vi "Value_Occurence_Analysis.vi"(3 "Average Numeric Values?":bool, 4 "Tolerance":dbl=1.0 format="%.2f", 5 "Precision (3)":string, 6 "String Array":string[](array[string])) -> (0 "Numeric Array?":bool, 1 "St Dev":string, 2 "Output String":string)   [LabVIEW 2020]
uses:
  <vilib>/Analysis/NI_AALBase.lvlib
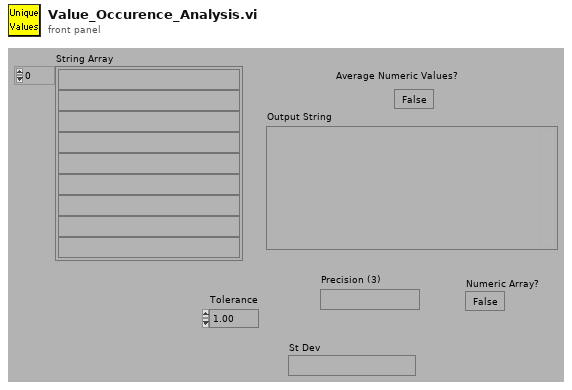
[diagram p1: front panel]
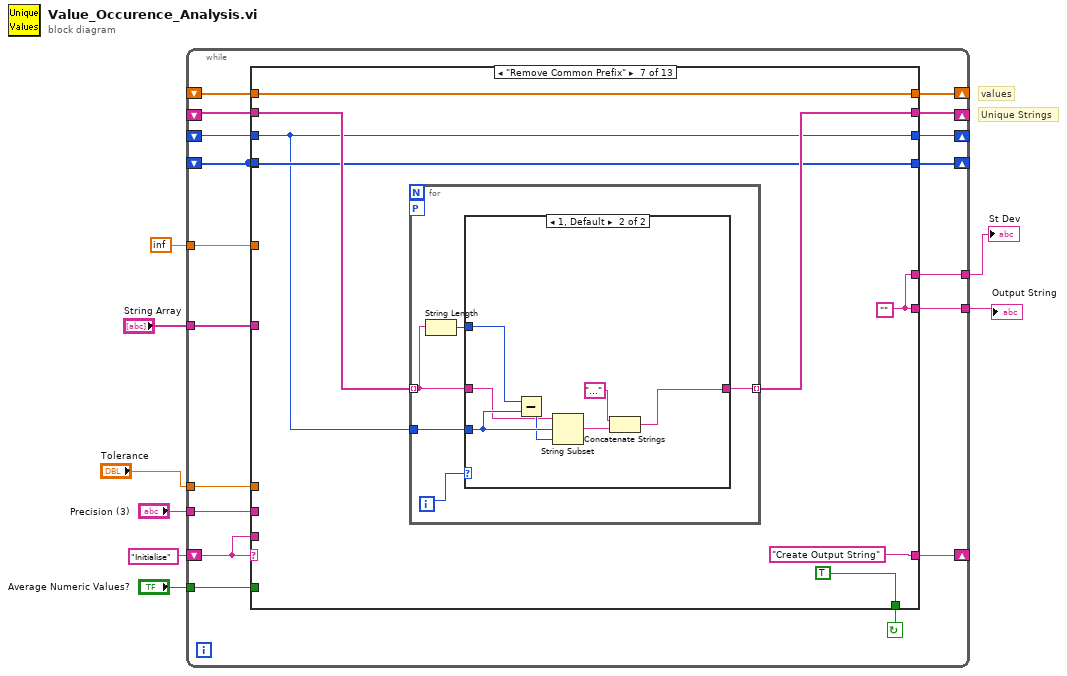
[diagram p0: block diagram]
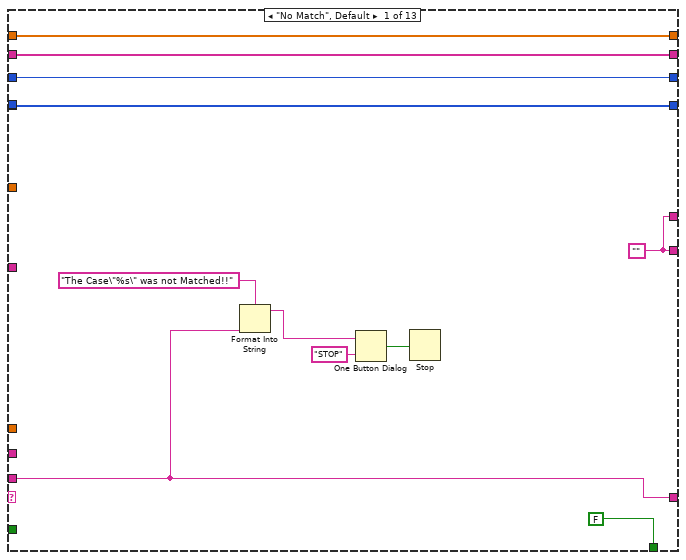
[diagram p2: hidden frame]
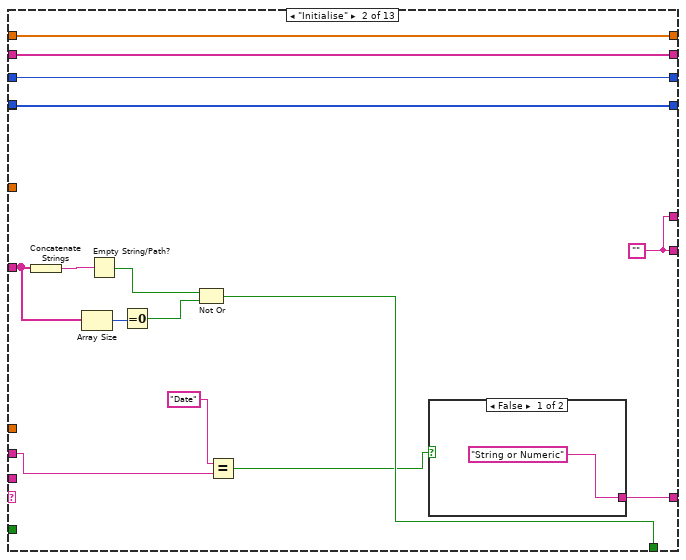
[diagram p3: hidden frame]
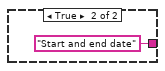
[diagram p4: hidden frame]
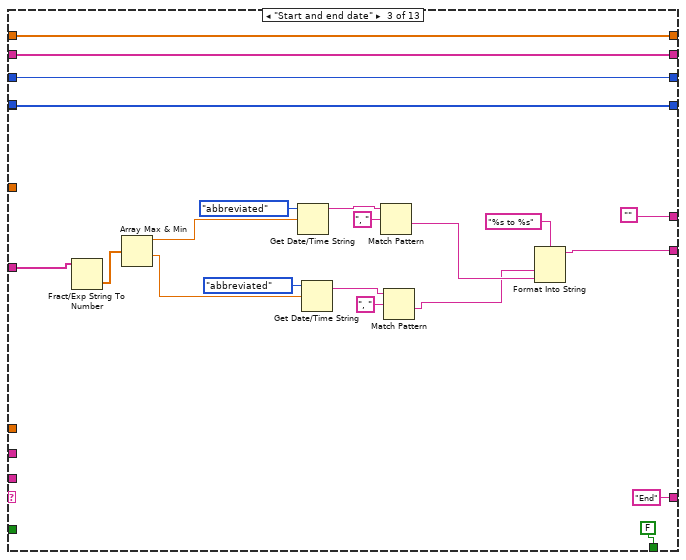
[diagram p5: hidden frame]
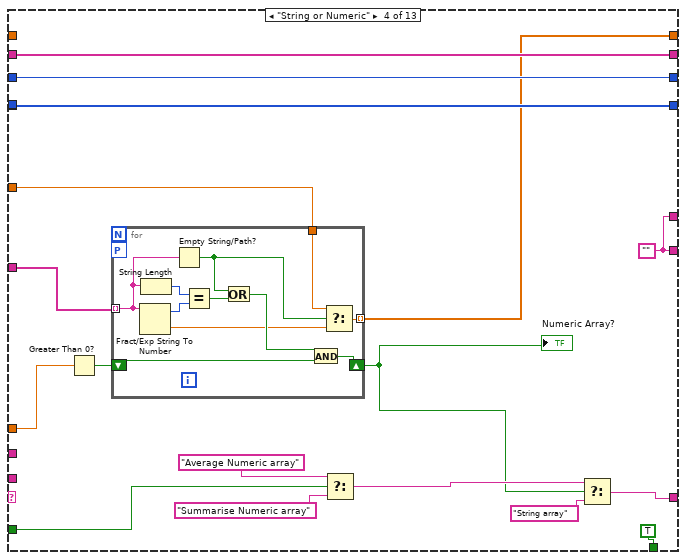
[diagram p6: hidden frame]
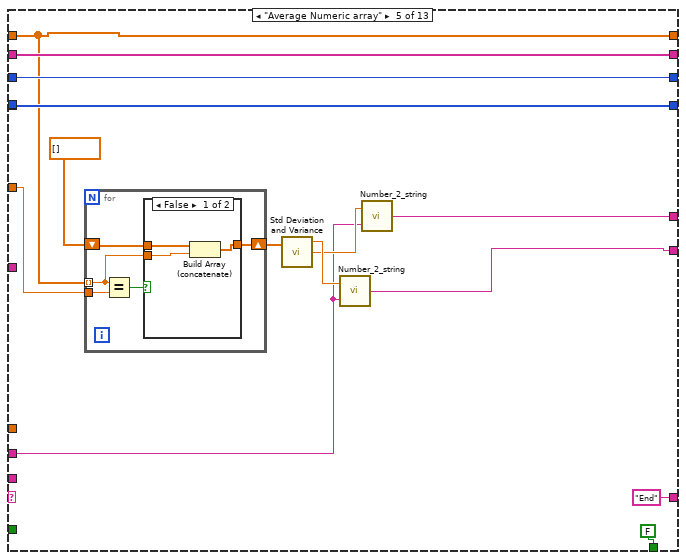
[diagram p7: hidden frame]
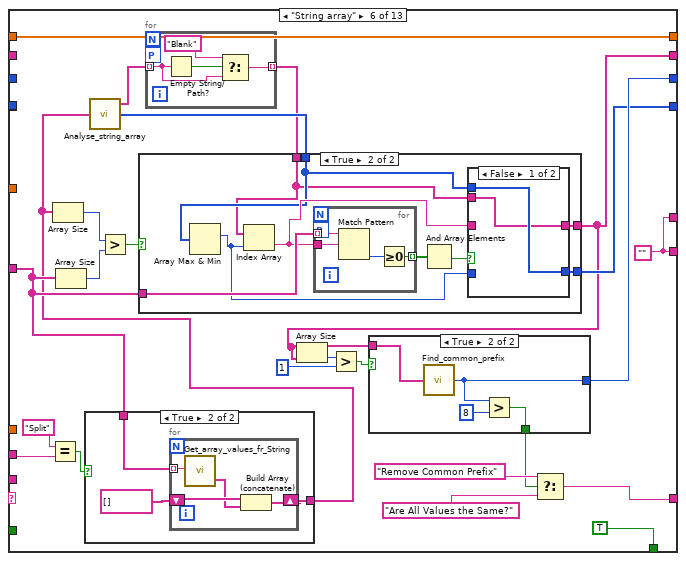
[diagram p9: hidden frame]
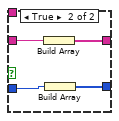
[diagram p12: hidden frame]
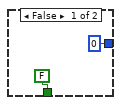
[diagram p13: hidden frame]
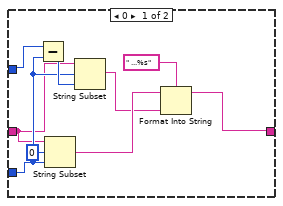
[diagram p14: hidden frame]
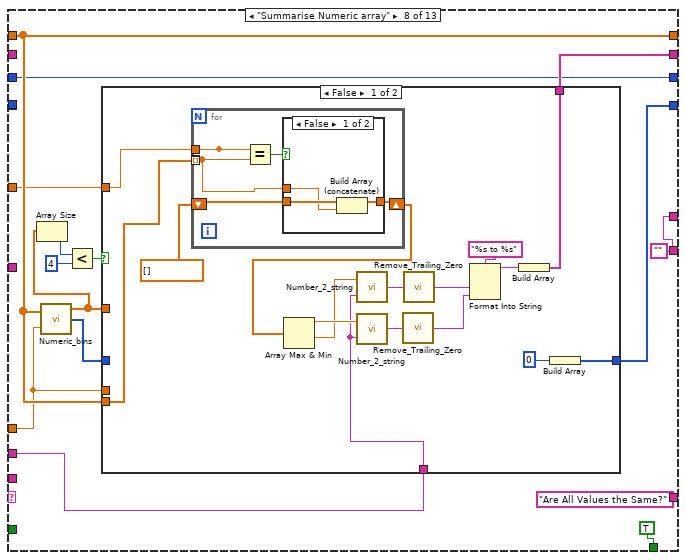
[diagram p15: hidden frame]
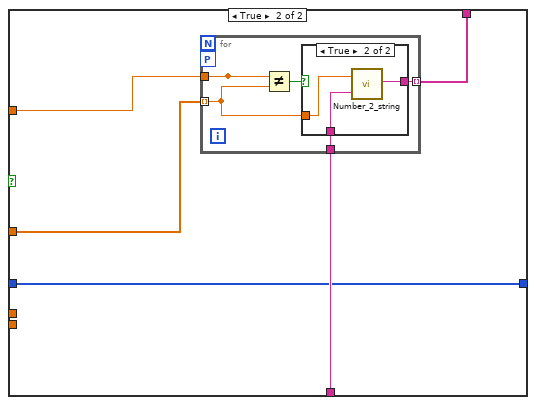
[diagram p17: hidden frame]
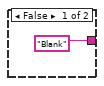
[diagram p18: hidden frame]
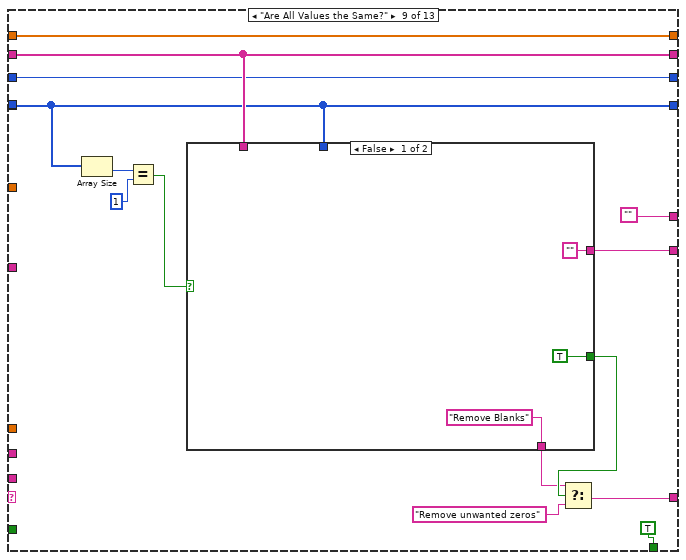
[diagram p19: hidden frame]
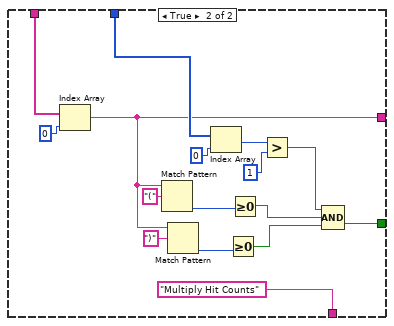
[diagram p20: hidden frame]
diagram:
  # "Unique Strings"
  # "values"
  n1 = while {
    shift-left: _ -> [w12]
    shift-right: [w13] -> _
    tunnel: [w14] -> w6
    shift-left: _ -> [w15]
    shift-right: [w16] -> _
    shift-left: _ -> [w17]
    shift-right: [w18] -> _
    tunnel: "Tolerance" -> [w19]
    shift-left: _ -> [w20]
    shift-right: [w24] -> _
    shift-left: "Initialise" -> [w21]
    shift-right: [w23] -> _
    tunnel: inf -> [w25]
    tunnel: "String Array" -> [w26]
    tunnel: "Average Numeric Values?" -> [w11]
    tunnel: "Precision (3)" -> [w10]
    tunnel: [w9] -> w2
    stop <- w22 continue-if-true
    n2 = case shown="\"Remove Common Prefix\"" w21 {
      tunnel: w26 -> [_ w47 w62 w88 _ w136 _ _ _ _ _ _ _]
      tunnel: w25 -> [_ _ _ w76 w111 _ _ w228 _ _ _ _ _]
      tunnel: [w32 w52 w71 w77 w110 w149 w196 w230 w286 w318 w350 w383 w401] -> w24
      tunnel: [w33 w49 "End" w91 "End" w144 "Create Output String" "Are All Values the Same?" w274 "End" "Remove unwanted zeros" "Create Output String" "Initialise"] -> w23
      tunnel: [FALSE w43 FALSE TRUE FALSE TRUE TRUE TRUE TRUE FALSE TRUE TRUE FALSE] -> w22
      tunnel: w21 -> [w33 _ _ _ _ _ _ _ _ _ _ _ _]
      tunnel: w20 -> [w32 w52 w71 _ w110 w149 w196 w230 w286 w318 w350 w383 w401]
      tunnel: w19 -> [_ _ _ w86 _ _ _ w229 _ _ _ _ _]
      tunnel: [w30 w51 w73 w89 w116 w134 w192 w227 w279 w315 w347 w382 w391] -> w18
      tunnel: w17 -> [w30 w51 w73 w89 w116 _ w192 _ w279 w315 w349 w382 w391]
      tunnel: w17 -> [_ _ _ _ _ _ _ _ _ _ _ _ _]
      tunnel: [w29 w50 w75 w90 w117 w133 w194 w231 w283 w317 w348 w379 w398] -> w16
      tunnel: w15 -> [w29 w50 w75 w90 w117 _ w193 _ w283 w317 w346 w380 w398]
      tunnel: [w27 w41 w65 w78 w112 w140 w190 w219 w281 w309 w344 w378 w397] -> w14
      tunnel: [w28 w42 w74 w84 w114 w148 w191 w222 w282 w316 w345 w381 w396] -> w13
      tunnel: w12 -> [w28 w42 w74 w84 w114 _ w191 w222 w282 w316 w345 w381 w396]
      tunnel: w11 -> [_ _ _ w83 _ _ _ _ _ _ _ _ _]
      tunnel: w10 -> [_ w40 _ _ w105 w132 _ w220 _ _ _ _ _]
      tunnel: [w27 w41 "" w78 w104 w140 w190 w219 "" "" w344 w378 ""] -> w9
      frame "No Match", Default {
        w27 = ""
        n3 = Format Into String(format string="The Case\"%s\" was not Matched!!" ("Format String"), w33) -> (resulting string=w36:string)  [unwired: 2 in, 1 out]
        n4 = One Button Dialog(message=w36, button name ("OK")="STOP") -> (true=w31:bool)
        n5 = Stop(stop? (T)=w31) -> ()
      }
      frame "Initialise" {
        w41 = ""
        n6 = Concatenate Strings(w47) -> (w48:string)
        n7 = Array Size(array=w47) -> (size(s)=w45:i32)
        n8 = Empty String/Path?(string/path=w48) -> (empty?=w46:bool)
        n9 = Equal To 0?(x=w45) -> (x = 0?=w44:bool)
        n10 = Not Or(1:w44, 2:w46) -> (0:w43:bool)
        n11 = Equal?(x="Date", y=w40) -> (x = y?=w38:bool)
        n12 = case shown="False" w38 {
          tunnel: ["String or Numeric" "Start and end date"] -> w49
          frame False {
          }
          frame True {
          }
        }
      }
      frame "Start and end date" {
        n13 = Fract/Exp String To Number(string=w62) -> (number=w61:dbl[])  [unwired: 4 out]
        n14 = Array Max & Min(array=w61) -> (max value=w70:dbl, min value=w67:dbl)  [unwired: 2 out]
        n15 = Get Date/Time String(date format (0)=enum16{"short", "long", "abbreviated"}."abbreviated", seconds (now)=w70) -> (date string=w59:string)  [unwired: 2 out]
        n16 = Get Date/Time String(date format (0)=enum16{"short", "long", "abbreviated"}."abbreviated", seconds (now)=w67) -> (date string=w57:string)  [unwired: 2 out]
        n17 = Match Pattern(string=w59, regular expression=", ") -> (after substring=w56:string)  [unwired: 4 out]
        n18 = Match Pattern(string=w57, regular expression=", ") -> (after substring=w55:string)  [unwired: 4 out]
        n19 = Format Into String(format string="%s to %s", w55, w56) -> (resulting string=w65:string)  [unwired: 2 in, 1 out]
      }
      frame "String or Numeric" {
        w78 = ""
        n20 = Greater Than 0?(x=w86) -> (x > 0?=w85:bool)
        n21 = for {
          tunnel: w88 -> [w94] mode=indexing
          shift-right: [w101] -> w79
          shift-left: w85 -> [w102]
          tunnel: [w98] -> w77 mode=indexing
          tunnel: w76 -> [w99]
          workers-P: _ -> [_]
          n22 = Fract/Exp String To Number(string=w94) -> (offset past number=w96:i32, number=w97:dbl)  [unwired: 3 out]
          n23 = String Length(string=w94) -> (length=w95:i32)
          n24 = Empty String/Path?(string/path=w94) -> (empty?=w100:bool)
          n25 = Equal?(x=w95, y=w96) -> (x = y?=w93:bool)
          n26 = Or(x=w100, y=w93) -> (x .or. y?=w103:bool)
          n27 = And(x=w103, y=w102) -> (x .and. y?=w101:bool)
          n28 = Select(t=w99, s=w100, f=w97) -> (s? t:f=w98:dbl)
        }
        "Numeric Array?" <- w79
        n29 = Select(t="Average Numeric array", s=w83, f="Summarise Numeric array") -> (s? t:f=w80:string)
        n30 = Select(t=w80, s=w79, f="String array") -> (s? t:f=w91:string)
      }
      frame "Average Numeric array" {
        n31 = for {
          shift-right: [w118] -> w108
          shift-left: dbl[] [] -> [w120]
          tunnel: w111 -> [w122]
          tunnel: w110 -> [w119] mode=indexing
          n32 = Equal?(x=w119, y=w122) -> (x = y?=w121:bool)
          n33 = case shown="False" w121 {
            tunnel: w120 -> [w125 w126]
            tunnel: w119 -> [w124 _]
            tunnel: [w123 w126] -> w118
            frame False {
              n34 = Build Array (concatenate)(w125, w124) -> (w123:dbl[])
            }
            frame True {
            }
          }
        }
        n35 = call <vilib>:"Std Deviation and Variance.vi"("X"=w108) -> ("mean"=w107:dbl, "standard deviation"=w106:dbl)  [unwired: 1 in, 1 out]
        n36 = call "Number_2_string.vi"("precision"=w105, "number"=w107) -> ("String"=w112:string)
        n37 = call "Number_2_string.vi"("precision"=w105, "number"=w106) -> ("String"=w104:string)
      }
      frame "String array" {
        w140 = ""
        n38 = Equal?(x="Split", y=w132) -> (x = y?=w129:bool)
        n39 = Array Size(array=w136) -> (size(s)=w138:i32)
        n40 = case shown="True" w129 {
          tunnel: [w155 w157] -> w130
          tunnel: w136 -> [w155 w156]
          frame False {
          }
          frame True {
            n41 = for {
              tunnel: w156 -> [w162] mode=indexing
              shift-right: [w160] -> w157
              shift-left: string[] [] -> [w161]
              n42 = call "Get_array_values_fr_String.vi"("String Value"=w162) -> ("String array"=w159:string[])  [unwired: 1 out]
              n43 = Build Array (concatenate)(w161, w159) -> (w160:string[])
            }
          }
        }
        n44 = Array Size(array=w130) -> (size(s)=w139:i32)
        n45 = call "Analyse_string_array.vi"("String array"=w130) -> ("Unique strings"=w128:string[], "Frequency"=w135:i32[])  [unwired: 1 out]
        n46 = Greater?(x=w139, y=w138) -> (0:w137:bool)
        n47 = for {
          tunnel: w128 -> [w153] mode=indexing
          tunnel: [w151] -> w127 mode=indexing
          workers-P: _ -> [_]
          n48 = Empty String/Path?(string/path=w153) -> (empty?=w154:bool)
          n49 = Select(t="Blank", s=w154, f=w153) -> (s? t:f=w151:string)
        }
        n50 = case shown="True" w137 {
          tunnel: w135 -> [w164 w166]
          tunnel: w127 -> [w163 w165]
          tunnel: w136 -> [_ w173]
          tunnel: [w163 w168] -> w133
          tunnel: [w164 w167] -> w134
          frame False {
          }
          frame True {
            n51 = Array Max & Min(array=w166) -> (max index (indices)=w170:i32)  [unwired: 3 out]
            n52 = Index Array(array=w165, index=w170) -> (element=w169:string)
            n53 = for {
              tunnel: w169 -> [w183]
              tunnel: w173 -> [w182] mode=indexing
              tunnel: [w180] -> w172 mode=indexing
              workers-P: _ -> [_]
              n54 = Match Pattern(string=w182, regular expression=w183) -> (offset past match=w181:i32)  [unwired: 4 out]
              n55 = Greater Or Equal To 0?(x=w181) -> (x >= 0?=w180:bool)
            }
            n56 = And Array Elements(Boolean array=w172) -> (logical AND=w171:bool)
            n57 = case shown="False" w171 {
              tunnel: w170 -> [_ w179]
              tunnel: w169 -> [_ w178]
              tunnel: [w174 w177] -> w168
              tunnel: [w175 w176] -> w167
              tunnel: w166 -> [w175 _]
              tunnel: w165 -> [w174 _]
              frame False {
              }
              frame True {
                n58 = Build Array(w178) -> (w177:string[])
                n59 = Build Array(w179) -> (w176:i32[])
              }
            }
          }
        }
        n60 = Array Size(array=w133) -> (size(s)=w143:i32)
        n61 = Greater?(x=w143, y=1) -> (0:w142:bool)
        n62 = case shown="True" w142 {
          tunnel: w133 -> [_ w189]
          tunnel: [0 ("Common Characters") w188] -> w148
          tunnel: [FALSE w187] -> w145
          frame False {
          }
          frame True {
            n63 = call "Find_common_prefix.vi"("Input Array"=w189) -> ("Common Characters"=w188:i32)
            n64 = Greater?(x=w188, y=8) -> (0:w187:bool)
          }
        }
        n65 = Select(t="Remove Common Prefix", s=w145, f="Are All Values the Same?") -> (s? t:f=w144:string)
      }
      frame "Remove Common Prefix" {
        w190 = ""
        n66 = for {
          tunnel: [w201] -> w194 mode=indexing
          tunnel: w193 -> [w199] mode=indexing
          tunnel: w191 -> [w200]
          workers-P: _ -> [_]
          i -> [w202]
          n67 = String Length(string=w199) -> (length=w198:i32)
          n68 = case shown="1, Default" w202 {
            tunnel: [w203 w215] -> w201
            tunnel: w199 -> [w207 w216]
            tunnel: w200 -> [w208 w218]
            tunnel: w198 -> [w209 w212]
            frame 0 {
              n69 = Subtract(x=w209, y=w208) -> (x-y=w210:i32)
              n70 = String Subset(string=w207, offset (0)=0, length (rest)=w208) -> (substring=w206:string)
              n71 = String Subset(string=w207, offset (0)=w208, length (rest)=w210) -> (substring=w205:string)
              n72 = Format Into String(format string=" ...%s" ("Format String"), initial string=w206, w205) -> (resulting string=w203:string)  [unwired: 1 in, 1 out]
            }
            frame 1, Default {
              n73 = Subtract(x=w212, y=w218) -> (x-y=w217:i32)
              n74 = String Subset(string=w216, offset (0)=w218, length (rest)=w217) -> (substring=w214:string)
              n75 = Concatenate Strings("..." ("Substring"), w214) -> (w215:string)
            }
          }
        }
      }
      frame "Summarise Numeric array" {
        w219 = ""
        n76 = call "Numeric_bins.vi"("Values"=w230, "Tolerance"=w229) -> ("Bin Centres"=w226:dbl[], "No of points in bins"=w221:i32[])  [unwired: 1 out]
        n77 = Array Size(array=w226) -> (size(s)=w225:i32)
        n78 = Less?(x=w225, y=4) -> (x < y?=w223:bool)
        n79 = case shown="False" w223 {
          tunnel: [w247 w263] -> w231
          tunnel: w230 -> [w241 _]
          tunnel: w229 -> [_ _]
          tunnel: w226 -> [_ w260]
          tunnel: w228 -> [w238 w261]
          tunnel: [w246 w259] -> w227
          tunnel: w220 -> [w242 w262]
          tunnel: w221 -> [_ w259]
          frame False {
            n80 = for {
              tunnel: [w250] -> _ mode=indexing
              tunnel: [w253] -> _ mode=indexing
              tunnel: w241 -> [w250] mode=indexing
              tunnel: w238 -> [w253]
              shift-right: [w251] -> w239
              shift-left: dbl[] [] -> [w252]
              n81 = Equal?(x=w253, y=w250) -> (x = y?=w254:bool)
              n82 = case shown="False" w254 {
                tunnel: w250 -> [w256 _]
                tunnel: w252 -> [w257 w258]
                tunnel: [w255 w258] -> w251
                frame False {
                  n83 = Build Array (concatenate)(w257, w256) -> (w255:dbl[])
                }
                frame True {
                }
              }
            }
            n84 = Array Max & Min(array=w239) -> (max value=w244:dbl, min value=w243:dbl)  [unwired: 2 out]
            n85 = call "Number_2_string.vi"("precision"=w242, "number"=w243) -> ("String"=w237:string)
            n86 = call "Number_2_string.vi"("precision"=w242, "number"=w244) -> ("String"=w236:string)
            n87 = call "Remove_Trailing_Zero.vi"("f"=w236) -> ("f 2"=w235:string)
            n88 = call "Remove_Trailing_Zero.vi"("f"=w237) -> ("f 2"=w234:string)
            n89 = Format Into String(format string="%s to %s" ("Format String"), w234, w235) -> (resulting string=w248:string)  [unwired: 2 in, 1 out]
            n90 = Build Array(w248) -> (w247:string[])
            n91 = Build Array(0) -> (w246:i32[])
          }
          frame True {
            n92 = for {
              tunnel: [w266] -> _ mode=indexing
              tunnel: [w267] -> w263 mode=indexing
              tunnel: w260 -> [w264] mode=indexing
              tunnel: w261 -> [w266]
              tunnel: w262 -> [w265]
              workers-P: _ -> [_]
              n93 = Not Equal?(x=w266, y=w264) -> (x != y?=w268:bool)
              n94 = case shown="True" w268 {
                tunnel: ["Blank" ("f") w272] -> w267
                tunnel: w264 -> [_ w271]
                tunnel: w265 -> [_ w270]
                frame False {
                }
                frame True {
                  n95 = call "Number_2_string.vi"("precision"=w270, "number"=w271) -> ("String"=w272:string)
                }
              }
            }
          }
        }
      }
      frame "Are All Values the Same?" {
        n96 = Array Size(array=w279) -> (size(s)=w284:i32)
        n97 = Equal?(x=w284, y=1) -> (x = y?=w280:bool)
        n98 = case shown="False" w280 {
          tunnel: w283 -> [_ w304]
          tunnel: ["" ("f") w290] -> w281
          tunnel: [TRUE w297] -> w276
          tunnel: w279 -> [_ w295]
          tunnel: ["Remove Blanks" "Multiply Hit Counts"] -> w275
          frame False {
          }
          frame True {
            n99 = Index Array(array=w304, index=0 ("Index")) -> (element=w290:string)
            n100 = Match Pattern(string=w290, regular expression="(") -> (offset past match=w301:i32)  [unwired: 4 out]
            n101 = Match Pattern(string=w290, regular expression=")") -> (offset past match=w300:i32)  [unwired: 4 out]
            n102 = Index Array(array=w295, index=0 ("Index")) -> (element=w294:i32)
            n103 = Greater Or Equal To 0?(x=w300) -> (x >= 0?=w299:bool)
            n104 = Greater Or Equal To 0?(x=w301) -> (x >= 0?=w298:bool)
            n105 = Greater?(x=w294, y=1) -> (0:w292:bool)
            n106 = Compound Arithmetic op=AND(w292, w298, w299) -> (w297:bool)
          }
        }
        n107 = Select(t=w275, s=w276, f="Remove unwanted zeros") -> (s? t:f=w274:string)
      }
      frame "Multiply Hit Counts" {
        n108 = Index Array(array=w317, index=0 ("Index")) -> (element=w312:string)
        n109 = Index Array(array=w315, index=0 ("Index")) -> (element=w311:i32)
        n110 = while {
          shift-right: [w333] -> _
          shift-left: w312 -> [w335]
          shift-right: [w324] -> w309
          shift-left: "" -> [w323]
          tunnel: w311 -> [w327]
          stop <- w331 continue-if-true
          n111 = Match Pattern(string=w335, regular expression="(") -> (before substring=w330:string, match substring=w329:string, after substring=w336:string)  [unwired: 2 out]
          n112 = Match Pattern(string=w336, regular expression=")") -> (before substring=w319:string, match substring=w325:string, after substring=w333:string)  [unwired: 2 out]
          n113 = Decimal String To Number(string=w319) -> (offset past number=w321:i32, number=w328:i32)  [unwired: 2 out]
          n114 = String Length(string=w319) -> (length=w322:i32)
          n115 = Match Pattern(string=w333, regular expression="(") -> (offset past match=w332:i32)  [unwired: 4 out]
          n116 = Equal?(x=w321, y=w322) -> (x = y?=w320:bool)
          n117 = case shown="True" w320 {
            tunnel: w328 -> [_ w343]
            tunnel: w327 -> [_ w342]
            tunnel: [w339 w340] -> w326
            tunnel: w319 -> [w339 _]
            frame False {
            }
            frame True {
              n118 = Multiply(x=w342, y=w343) -> (x*y=w341:i32)
              n119 = Number To Decimal String(number=w341) -> (decimal integer string=w340:string)  [unwired: 1 out]
            }
          }
          n120 = Greater Or Equal To 0?(x=w332) -> (x >= 0?=w331:bool)
          n121 = Concatenate Strings(w323, w330, w329, w326, w325) -> (w324:string)
        }
      }
      frame "Remove Blanks" {
        w344 = ""
        n122 = Empty String/Path?(string/path=w346) -> (empty?=w352:bool[])
        n123 = Or Array Elements(Boolean array=w352) -> (logical OR=w351:bool)
        n124 = case shown="True" w351 {
          tunnel: w346 -> [w355 w357]
          tunnel: w349 -> [w356 w362]
          tunnel: [w355 w359] -> w348
          tunnel: [w356 w358] -> w347
          frame False {
          }
          frame True {
            n125 = for {
              shift-right: [w366] -> w359
              shift-left: string[] [] -> [w367]
              shift-right: [w365] -> w358
              shift-left: i32[] [] -> [w368]
              tunnel: w357 -> [w363] mode=indexing
              tunnel: w362 -> [w364] mode=indexing
              n126 = Empty String/Path?(string/path=w363) -> (empty?=w369:bool)
              n127 = case shown="False" w369 {
                tunnel: w368 -> [w375 w376]
                tunnel: w367 -> [w374 w377]
                tunnel: [w373 w377] -> w366
                tunnel: [w372 w376] -> w365
                tunnel: w363 -> [w371 _]
                tunnel: w364 -> [w370 _]
                frame False {
                  n128 = Build Array (concatenate)(w374, w371) -> (w373:string[])
                  n129 = Build Array (concatenate)(w375, w370) -> (w372:i32[])
                }
                frame True {
                }
              }
            }
          }
        }
      }
      frame "Remove unwanted zeros" {
        w378 = ""
        n130 = for {
          tunnel: w380 -> [w386] mode=indexing
          tunnel: [w387] -> w379 mode=indexing
          workers-P: _ -> [_]
          n131 = call "Remove_Trailing_Zero.vi"("f"=w386) -> ("f 2"=w387:string)
        }
      }
      frame "Create Output String" {
        n132 = Array Size(array=w391) -> (size(s)=w390:i32)
        n133 = Equal?(x=w391, y=1) -> (x = y?=w394:bool[])
        n134 = Equal?(x=w390, y=1) -> (x = y?=w388:bool)
        n135 = And Array Elements(Boolean array=w394) -> (logical AND=w393:bool)
        n136 = case shown="True" w388 {
          tunnel: w398 -> [w410 w428]
          tunnel: [w404 w426] -> w397
          tunnel: w393 -> [w403 _]
          tunnel: w391 -> [w402 _]
          frame False {
            n137 = for {
              shift-right: [w415] -> w408
              shift-left: "" -> [w416]
              tunnel: w410 -> [w414] mode=indexing
              tunnel: w402 -> [w413] mode=indexing
              tunnel: w403 -> [w412]
              n138 = case shown="False" w412 {
                tunnel: w416 -> [w421 w425]
                tunnel: [w420 w424] -> w415
                tunnel: w414 -> [w419 w423]
                tunnel: w413 -> [w418 _]
                frame False {
                  n139 = Format Into String(format string="%s (%d);  " ("Format String"), initial string=w421, w419, w418) -> (resulting string=w420:string)  [unwired: 1 in, 1 out]
                }
                frame True {
                  n140 = Format Into String(format string="%s;  " ("Format String"), initial string=w425, w423) -> (resulting string=w424:string)  [unwired: 1 in, 1 out]
                }
              }
            }
            n141 = String Length(string=w408) -> (length=w406:i32)
            n142 = Subtract(x=w406, y=2) -> (x-y=w405:i32)
            n143 = String Subset(string=w408, offset (0)=0, length (rest)=w405) -> (substring=w404:string)
          }
          frame True {
            n144 = Index Array(array=w428, index=0) -> (element=w426:string)
          }
        }
      }
    }
  }
  "Output String" <- w6
  "St Dev" <- w2
